vi "roboRIO v1.0 Shutdown Encoder.vi"(8 "error in (no error)":errorcluster, 10 "Channel":T1, 11 "myRIO Ref In":T2) -> (0 "error out":errorcluster, 3 "myRIO Ref Out":T2)   [LabVIEW 2021]
uses:
  <vilib>/myRIO/Common/Instrument Driver Framework/Utilities/typedefs/myRIO v1.0 Reference.ctl
  <vilib>/myRIO/Common/Instrument Driver Framework/Utilities/typedefs/Generic FPGA Reference.ctl
  <vilib>/myRIO/Common/Instrument Driver Framework/myRIO v1.0/Encoder/typedefs/Encoder Channels Enum.ctl
  <vilib>/myRIO/Common/Instrument Driver Framework/myRIO v1.0/Encoder/typedefs/Encoder Config Manager Action Enum.ctl
  <vilib>/myRIO/Common/Instrument Driver Framework/roboRIO v1.0/Encoder/typedefs/roboRIO Encoder Channels FPGA Reference.ctl
  <vilib>/rvi/errors/niLvFpgaAdjustHostInterfaceError.vi
  <vilib>/rvi/interface/nirviReadWriteControl/nirviReadWriteControl.xnode
  NiFpgaLv.dll
  <vilib>/rvi/interface/Simulation/niFpgaSimulationCallBeginRW.vi
panel:
  # "This VI turns off the specified Encoder channel and zeroes out all of its registers."
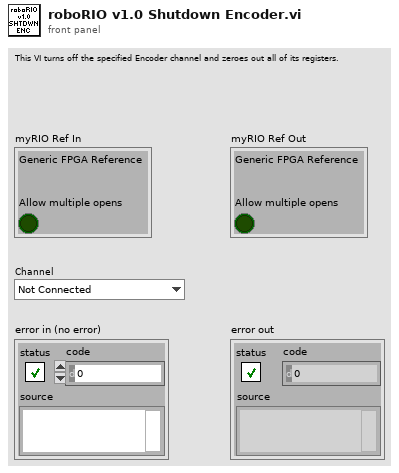
[diagram p1: front panel]
types:
  T1 = typedef "Encoder Channels Enum.ctl" = enum16{"Not Connected", "C/ENC0", "C/ENC1", "A/ENC", "A/ENC0", "A/ENC1", "A/ENC2", "A/ENC3", "A/ENC4", "A/ENC5", "A/ENC6", "A/ENC7", "A/ENC8", "A/ENC9", "B/ENC", "B/ENC0", "B/ENC1", "B/ENC2", "B/ENC3", "B/ENC4", "B/ENC5", "B/ENC6", "B/ENC7", "B/ENC8", "B/ENC9", "DIO/ENC0", "DIO/ENC1", "DIO/ENC2", "DIO/ENC3", "DIO/ENC4"}
  T2 = typedef "myRIO v1.0 Reference.ctl" = cluster{"Generic FPGA Reference":T3, "Allow multiple opens":bool}
  T3 = typedef "Generic FPGA Reference.ctl" = refnum<k20>
  T4 = typedef "Encoder Config Manager Action Enum.ctl" = enum16{"Do Nothing", "Store", "Clear"}
  T5 = typedef "roboRIO Encoder Channels FPGA Reference.ctl" = refnum<k20>
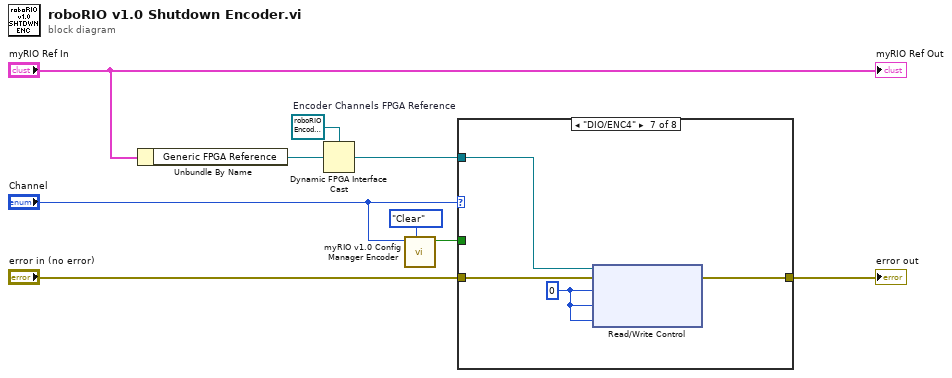
[diagram p0: block diagram]
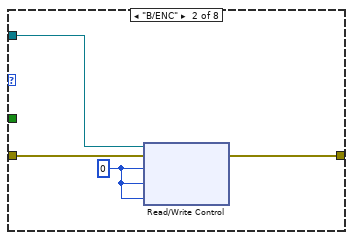
[diagram p3: hidden frame]
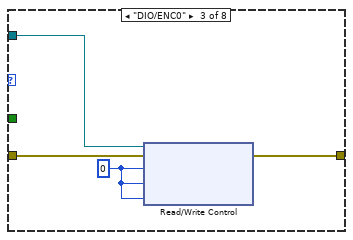
[diagram p4: hidden frame]
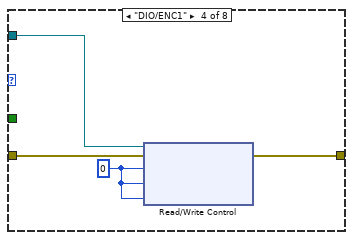
[diagram p5: hidden frame]
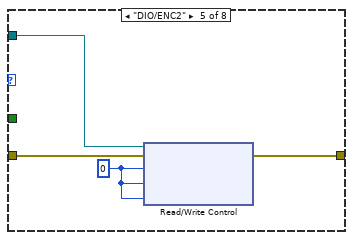
[diagram p6: hidden frame]
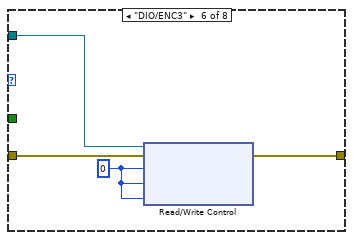
[diagram p7: hidden frame]
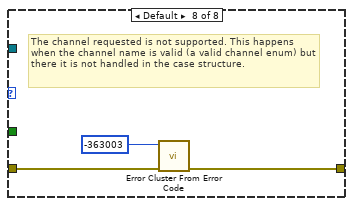
[diagram p8: hidden frame]
diagram:
  w9 = T5 refnum  # Encoder Channels FPGA Reference
  n1 = Unbundle By Name("myRIO Ref In") -> ("Generic FPGA Reference"=w5:T3)
  n2 = Dynamic FPGA Interface Cast(Session In=w9, Type=w5) -> (Session Out=w8:T5)
  n3 = call <vilib>:"myRIO v1.0 Config Manager Encoder.vi"("Action"=Encoder_Config_Manager_Action_Enum."Clear", "Encoder Channel"="Channel") -> ("Success?"=w1:bool)  [unwired: 9 in]
  n4 = case shown="\"DIO/ENC4\"" "Channel" {
    tunnel: "error in (no error)" -> [w10 w13 w17 w21 w25 w29 w33 w35]
    tunnel: [w10 w11 w15 w19 w23 w27 w31 w36] -> w6
    tunnel: w8 -> [_ w14 w18 w22 w26 w30 w34 _]
    tunnel: w1 -> [_ _ _ _ _ _ _ _]
    frame "Not Connected" {
    }
    frame "B/ENC" {
      w12 = u8 0 ("ENC.C_0.CNFG")
      n5 = xnode "Read/Write Control"("FPGA VI Reference In"=w14, "error in"=w13, "ENC.B.CNFG"=w12, "ENC.B.CNTR"=w12, "ENC.B.STAT"=w12) -> ("error out"=w11:errorcluster)  [unwired: 1 out]
    }
    frame "DIO/ENC0" {
      w16 = u8 0 ("ENC.C_0.CNFG")
      n6 = xnode "Read/Write Control"("FPGA VI Reference In"=w18, "error in"=w17, "ENC.DIO_0.CNFG"=w16, "ENC.DIO_0.CNTR"=w16, "ENC.DIO_0.STAT"=w16) -> ("error out"=w15:errorcluster)  [unwired: 1 out]
    }
    frame "DIO/ENC1" {
      w20 = u8 0 ("ENC.C_0.CNFG")
      n7 = xnode "Read/Write Control"("FPGA VI Reference In"=w22, "error in"=w21, "ENC.DIO_1.CNFG"=w20, "ENC.DIO_1.CNTR"=w20, "ENC.DIO_1.STAT"=w20) -> ("error out"=w19:errorcluster)  [unwired: 1 out]
    }
    frame "DIO/ENC2" {
      w24 = u8 0 ("ENC.C_0.CNFG")
      n8 = xnode "Read/Write Control"("FPGA VI Reference In"=w26, "error in"=w25, "ENC.DIO_2.CNFG"=w24, "ENC.DIO_2.CNTR"=w24, "ENC.DIO_2.STAT"=w24) -> ("error out"=w23:errorcluster)  [unwired: 1 out]
    }
    frame "DIO/ENC3" {
      w28 = u8 0 ("ENC.C_0.CNFG")
      n9 = xnode "Read/Write Control"("FPGA VI Reference In"=w30, "error in"=w29, "ENC.DIO_3.CNFG"=w28, "ENC.DIO_3.CNTR"=w28, "ENC.DIO_3.STAT"=w28) -> ("error out"=w27:errorcluster)  [unwired: 1 out]
    }
    frame "DIO/ENC4" {
      w32 = u8 0 ("ENC.C_0.CNFG")
      n10 = xnode "Read/Write Control"("FPGA VI Reference In"=w34, "error in"=w33, "ENC.DIO_4.CNFG"=w32, "ENC.DIO_4.CNTR"=w32, "ENC.DIO_4.STAT"=w32) -> ("error out"=w31:errorcluster)  [unwired: 1 out]
    }
    frame Default {
      # "The channel requested is not supported. This happens when the channel name is valid (a valid channel enum) but there it is not handled in the case structure."
      n11 = call <vilib>:"Error Cluster From Error Code.vi"("error in (no error)"=w35, "error code (0)"=-363003) -> ("error out"=w36:errorcluster)  [unwired: 7 in]
    }
  }
  "error out" <- w6
  "myRIO Ref Out" <- "myRIO Ref In"
